vi "Create Name.vi"(8 "error in (no error)":errorcluster) -> (0 "error out":errorcluster, 2 "Name":string)   [LabVIEW 2015, in "navX Library v3.lvlib" / "navX - Interface.lvclass"]
uses:
  navX - Interface.lvclass
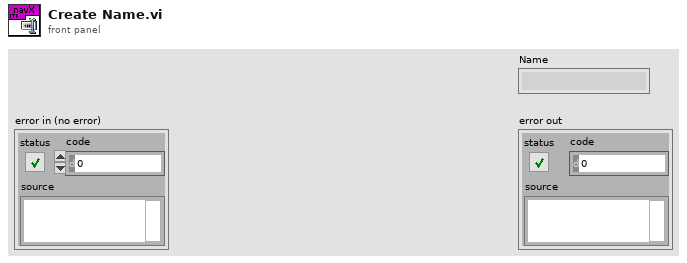
[diagram p1: front panel]
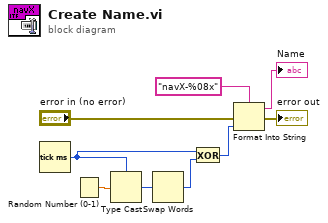
[diagram p0: block diagram]
diagram:
  n1 = Tick Count (ms)() -> (millisecond timer value=w3:u32)
  n2 = Random Number (0-1)() -> (number: 0 to 1=w4:dbl)
  n3 = Type Cast(type=w3, x=w4) -> (*(type *) &x=w2:u32)
  n4 = Swap Words(1:w2) -> (0:w1:u32)
  n5 = Exclusive Or(1:w1, 2:w3) -> (0:w5:u32)
  n6 = Format Into String(format string="navX-%08x" ("name (unnamed)"), error in="error in (no error)", w5) -> (resulting string=→"Name":string, error out=→"error out":errorcluster)  [unwired: 1 in]
